vi "Reset.vi"(8 "错误输入（无错误）":errorcluster, 11 "VISA资源名称":refnum<visa-resource-name>) -> (0 "错误输出":errorcluster, 3 "VISA资源名称输出":refnum<visa-resource-name>)   [LabVIEW 2018]
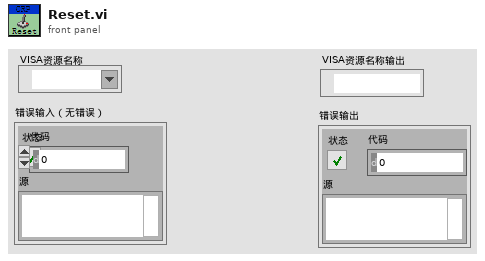
[diagram p1: front panel]
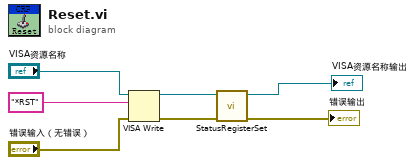
[diagram p0: block diagram]
diagram:
  n1 = VISA Write(VISA resource name="VISA资源名称", write buffer="*RST" ("SCPI字符串"), error in (no error)="错误输入（无错误）") -> (VISA resource name out=w4:refnum<visa-resource-name>, error out=w3:errorcluster)  [unwired: 1 out]
  n2 = call "StatusRegisterSet.vi"("错误输入（无错误）"=w3, "VISA引用句柄输入"=w4) -> ("错误输出"=→"错误输出":errorcluster, "VISA引用句柄输出"=→"VISA资源名称输出":refnum<visa-resource-name>)  [unwired: 8 in]
